vi "MeasurementConfigToJSON.vi"(8 "ErrorIn":errorcluster, 10 "MeasurementConfig":T1={"Frequency"=100, "Resolution[b]"=16, "AccelFSRange"=enum."+/-2g", "GyroFSRange"=enum."+/-250dps"} {"Resolution[b]" min=4 max=16 step=1; "Frequency" min=1 max=10000000 step=1}, 11 "JSONIn":refnum<class "JSON Object.lvclass">) -> (0 "ErrorOut":errorcluster, 2 "JSONMeasurementConfigPretty":string, 3 "JSONOut":refnum<class "JSON Object.lvclass">)   [LabVIEW 2016]
doc: "Convert MeasurementConfig to JSON. Return also JSONOut to combine with other JSON objects."
uses:
  FallSensor/MeasurementConfig.ctl
  FallSensor/Measurement/AccelFSRange.ctl
  FallSensor/Measurement/GyroFSRange.ctl
  <vilib>/addons/JSON API/JSON Object/JSON Object.lvclass
  D:/Programy/National Instruments/LabVIEW 2016/vi.lib/addons/JSON API/JSON Value/JSON Value.lvclass
  <vilib>/addons/JSON API/JSON Object/Set Object Item by name.vi
  <vilib>/addons/JSON API/JSON Value/Get as JSON string.vi
  <vilib>/addons/JSON API/JSON Scalar/JSON Scalar.lvclass
  <vilib>/addons/JSON API/JSON Scalar/Set U32.vi
  <vilib>/addons/JSON API/JSON Value/Get as JSON string (pretty).vi
  <vilib>/addons/JSON API/JSON Value/Get Item by name array.vi
  <vilib>/addons/JSON API/JSON Value/JSON Value.lvclass
  <vilib>/addons/JSON API/Get Polymorphic/JSON GetSet.lvlib
panel:
  out "JSONMeasurementConfigRaw":string
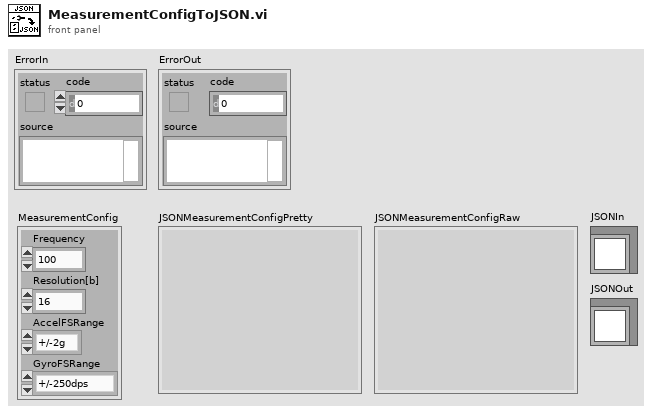
[diagram p1: front panel]
types:
  T1 = typedef "MeasurementConfig.ctl" = cluster{"Frequency":u32, "Resolution[b]":u32, "AccelFSRange":T2, "GyroFSRange":T3}
  T2 = typedef "AccelFSRange.ctl" = enum16{"+/-2g", "+/-4g", "+/-8g", "+/-16g"}
  T3 = typedef "GyroFSRange.ctl" = enum16{"+/-250dps", "+/-500dps", "+/-1000dps", "+/-2000dps"}
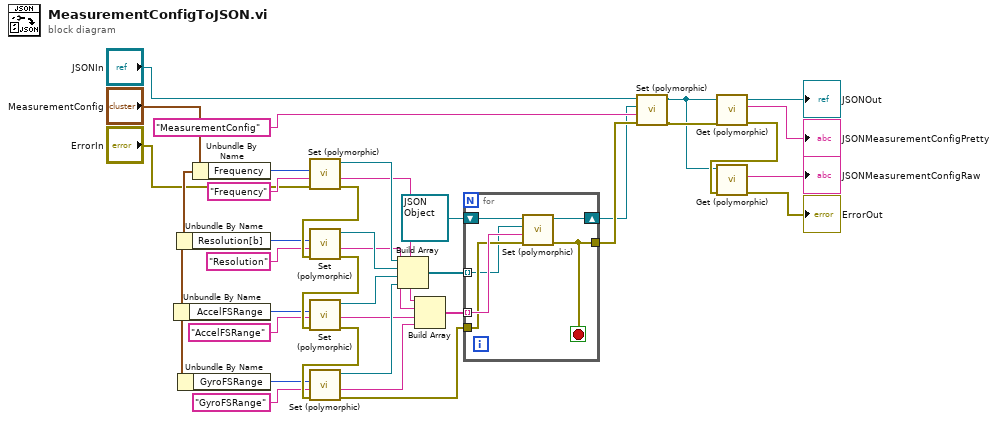
[diagram p0: block diagram]
diagram:
  n1 = Unbundle By Name("MeasurementConfig") -> ("AccelFSRange"=w11:T2)
  n2 = Unbundle By Name("MeasurementConfig") -> ("Resolution[b]"=w12:u32)
  n3 = Unbundle By Name("MeasurementConfig") -> ("GyroFSRange"=w10:T3)
  n4 = Unbundle By Name("MeasurementConfig") -> ("Frequency"=w31:u32)
  n5 = call-poly <vilib>:"Set (polymorphic).vi"("error in (no error)"="ErrorIn", "Numeric"=w31) -> ("error out"=w26:errorcluster, "JSON Scalar out"=w30:refnum<class "JSON Scalar.lvclass">)  [unwired: 8 in]
  n6 = call-poly <vilib>:"Set (polymorphic).vi"("error in (no error)"=w26, "Numeric"=w12) -> ("error out"=w25:errorcluster, "JSON Scalar out"=w29:refnum<class "JSON Scalar.lvclass">)  [unwired: 8 in]
  n7 = call-poly <vilib>:"Set (polymorphic).vi"("error in (no error)"=w25, "Numeric"=w11) -> ("error out"=w24:errorcluster, "JSON Scalar out"=w28:refnum<class "JSON Scalar.lvclass">)  [unwired: 8 in]
  n8 = call-poly <vilib>:"Set (polymorphic).vi"("error in (no error)"=w24, "Numeric"=w10) -> ("error out"=w16:errorcluster, "JSON Scalar out"=w27:refnum<class "JSON Scalar.lvclass">)  [unwired: 8 in]
  n9 = Build Array(w30, w29, w28, w27) -> (w22:refnum<class "JSON Scalar.lvclass">[])
  n10 = Build Array("Frequency" ("name"), "Resolution" ("name"), "AccelFSRange" ("name"), "GyroFSRange" ("name")) -> (w17:string[])
  n11 = for {
    shift-right: [w33] -> w13
    shift-left: refnum<class "JSON Object.lvclass"> refnum ("JSON Object out") -> [w37]
    tunnel: w22 -> [w34] mode=indexing
    tunnel: w17 -> [w36] mode=indexing
    tunnel: w16 -> [w35]
    tunnel: [w32] -> w14
    stop <- w32 stop-if-true
    n12 = call-poly <vilib>:"Set (polymorphic).vi"("error in (no error)"=w35, "name"=w36, "Value"=w34, "JSON Object in"=w37) -> ("error out"=w32:errorcluster, "JSON Object out"=w33:refnum<class "JSON Object.lvclass">)  [unwired: 5 in, 1 out]
  }
  n13 = call-poly <vilib>:"Set (polymorphic).vi"("error in (no error)"=w14, "name"="MeasurementConfig", "Value"=w13, "JSON Object in"="JSONIn") -> ("error out"=w7:errorcluster, "JSON Object out"=w2:refnum<class "JSON Object.lvclass">)  [unwired: 5 in, 1 out]
  "JSONOut" <- w2
  n14 = call-poly <vilib>:"Get (polymorphic).vi"("error in (no error)"=w7, "JSON Value in"=w2) -> ("error out"=w4:errorcluster, "<JSON>"=→"JSONMeasurementConfigPretty":string)  [unwired: 8 in]
  n15 = call-poly <vilib>:"Get (polymorphic).vi"("error in (no error)"=w4, "JSON Value in"=w2) -> ("error out"=→"ErrorOut":errorcluster, "<JSON>"=→"JSONMeasurementConfigRaw":string)  [unwired: 8 in]
